vi "JSON format Test.vi"() -> ()   [LabVIEW 2020, in "JSONtext.lvlib"]
uses:
  <vilib>/JDP Science/JSONtext/JSONtext.lvlib
panel:
  out "error out":errorcluster
  out "length":i32
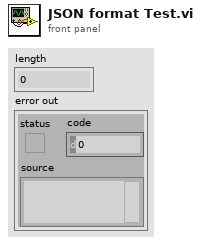
[diagram p1: front panel]
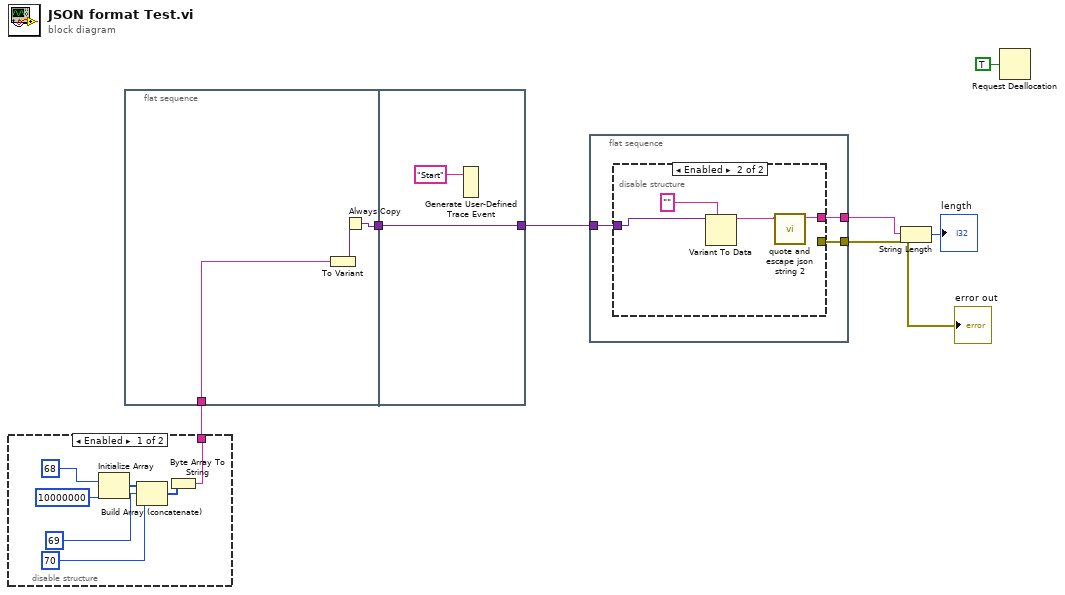
[diagram p0: block diagram]
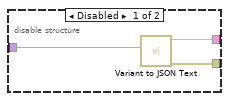
[diagram p3: hidden frame]
diagram:
  n1 = disable-structure shown="Enabled" {
    disable-tunnel: [w10 _] -> w1
    frame Enabled {
      n2 = Initialize Array(u8 68 ("element"), 10000000 ("dimension size")) -> (w12:u8[])
      n3 = Build Array (concatenate)(w12, u8 69 ("element"), u8 70 ("element")) -> (w11:u8[])
      n4 = Byte Array To String(unsigned byte array=w11) -> (string=w10:string)
    }
    frame Disabled {
    }
  }
  n5 = flat-sequence {
    tunnel: [w17] -> w3
    tunnel: w1 -> [w15]
    tunnel: [w19] -> w2
    tunnel: w3 -> [w19]
    frame #0 {
      n6 = To Variant(anything=w15) -> (Variant=w16:variant)
      n7 = Always Copy(1:w16) -> (0:w17:variant)
    }
    frame #1 {
      n8 = Generate User-Defined Trace Event(2:"Start" ("trace string")) -> ()  [unwired: 1 in]
    }
  }
  n9 = flat-sequence {
    tunnel: w2 -> [w20]
    tunnel: [w22] -> w7
    tunnel: [w21] -> w5
    frame #0 {
      n10 = disable-structure shown="Enabled" {
        disable-tunnel: [w25 w26] -> w22
        disable-tunnel: [w24 _] -> w21
        disable-tunnel: w20 -> [w23 w28]
        frame Disabled {
          n11 = call <vilib>:"Variant to JSON Text.vi"("Variant"=w23) -> ("error out"=w24:errorcluster, "<JSON>"=w25:string)  [unwired: 8 in, 1 out]
        }
        frame Enabled {
          n12 = Variant To Data(type="", Variant=w28) -> (data=w27:string)  [unwired: 1 in, 1 out]
          n13 = call <vilib>:"quote and escape json string 2.vi"("base string"=w27) -> ("String out"=w26:string)  [unwired: 10 in]
        }
      }
    }
  }
  n14 = String Length(string=w7) -> (length=→"length":i32)
  n15 = Request Deallocation(TRUE ("flag")) -> ()
  "error out" <- w5
